vi "Get UpdateSytle Event.vi"(8 "error in (no error)":errorcluster, 11 "Canvas in":refnum<class "Canvas.lvclass">) -> (0 "error out":errorcluster, 2 "UpdateSytle Event":refnum<user-event>, 3 "Canvas out":refnum<class "Canvas.lvclass">)   [LabVIEW 2015, in "Canvas.lvclass"]
uses:
  Canvas.lvclass
  Graphic/Ctls/Style.ctl
  Canvas.lvclass/Canvas.ctl
  Graphic/Graphic.lvclass
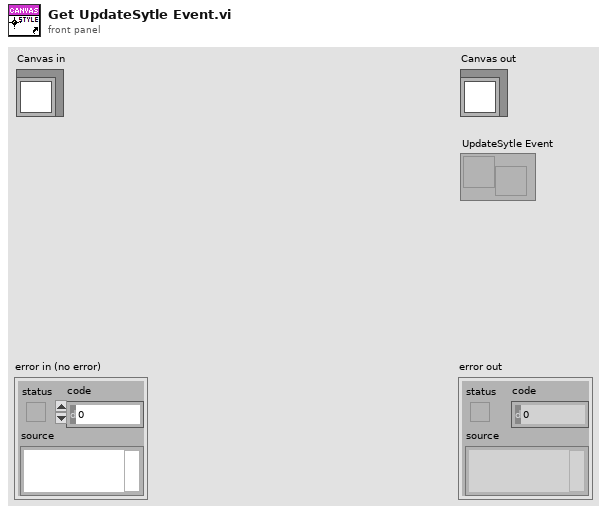
[diagram p1: front panel]
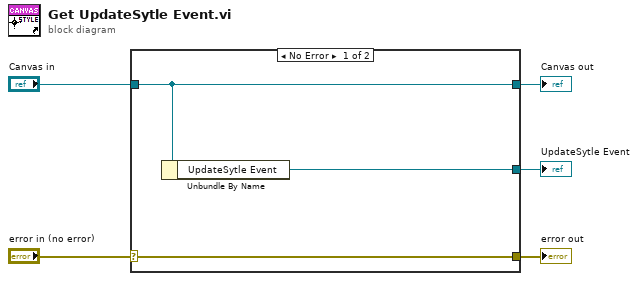
[diagram p0: block diagram]
diagram:
  n1 = case shown="No Error" "error in (no error)" {
    selector: "error in (no error)" -> [w8 w9]
    tunnel: [w8 w9] -> w4
    tunnel: [w7 w10] -> w2
    tunnel: "Canvas in" -> [w7 w10]
    tunnel: [w6 _] -> w1
    frame No Error {
      n2 = Unbundle By Name(w7) -> ("UpdateSytle Event"=w6:refnum<user-event>)
    }
    frame Error {
    }
  }
  "error out" <- w4
  "Canvas out" <- w2
  "UpdateSytle Event" <- w1
